vi "DCON-ParseDO.vi"(7 "Read Buffer":string) -> (8 "Boolean array":bool[](array[boolean]))   [LabVIEW 2011]
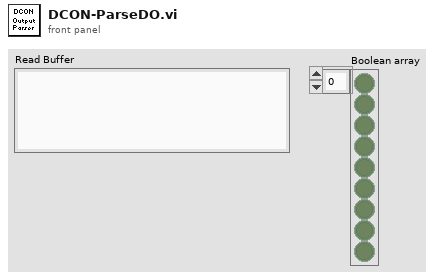
[diagram p1: front panel]
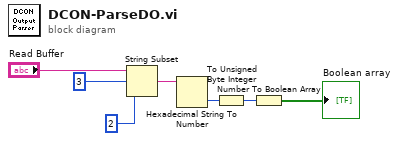
[diagram p0: block diagram]
diagram:
  n1 = String Subset(string="Read Buffer", offset (0)=3, length (rest)=2 ("length (rest)")) -> (substring=w5:string)
  n2 = Hexadecimal String To Number(string=w5) -> (number=w4:u32)  [unwired: 2 in, 1 out]
  n3 = To Unsigned Byte Integer(number=w4) -> (unsigned 8bit integer=w1:u8)
  n4 = Number To Boolean Array(number=w1) -> (Boolean array=→"Boolean array":bool[])
